vi "Size.vi"(7 "VI":refnum<vi>, 8 "Error":errorcluster, 9 "WkSpace":T1, 11 "(FPSZ)":refnum<class "FPSZ.lvclass">) -> (0 "Error Out":errorcluster, 3 "(FPSZ) Out":refnum<class "FPSZ.lvclass">, 5 "VI Out":refnum<vi>)   [LabVIEW 2020, in "FPSZ.lvclass"]
uses:
  FPSZ.lvclass
  <vilib>/Utility/miscctls.llb/LVRectTypeDef.ctl
  FPSZ.lvclass/FPSZ.ctl
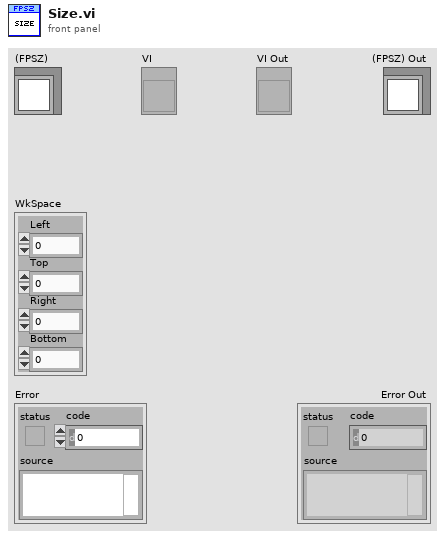
[diagram p1: front panel]
types:
  T1 = typedef "LVRectTypeDef.ctl" = cluster{"Left":i16, "Top":i16, "Right":i16, "Bottom":i16}
  T2 = typedef "LVPositionTypeDef.ctl" = cluster{"Left":i32, "Top":i32}
  T3 = typedef "LVBoundsTypeDef.ctl" = cluster{"Width":u32, "Height":u32}
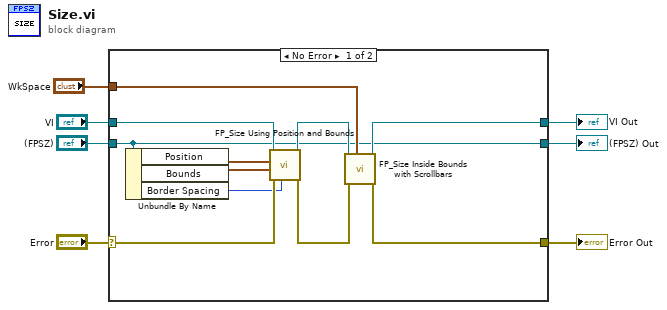
[diagram p0: block diagram]
diagram:
  n1 = case shown="No Error" "Error" {
    selector: "Error" -> [w18 w21]
    tunnel: [w12 w21] -> w6
    tunnel: [w8 w20] -> w4
    tunnel: "(FPSZ)" -> [w8 w20]
    tunnel: "VI" -> [w17 w19]
    tunnel: [w13 w19] -> w2
    tunnel: "WkSpace" -> [w14 _]
    frame No Error {
      n2 = Unbundle By Name(w8) -> ("Position"=w10:T2, "Bounds"=w9:T3, "Border Spacing"=w11:i16)
      n3 = call "FP_Size Using Position and Bounds.vi"("Border Spacing"=w11, "Error"=w18, "Bounds"=w9, "Position"=w10, "VI"=w17) -> ("Error Out"=w15:errorcluster, "VI Out"=w16:refnum<vi>)  [unwired: 4 in, 1 out]
      n4 = call "FP_Size Inside Bounds with Scrollbars.vi"("WkSpace"=w14, "Error"=w15, "VI"=w16) -> ("Error Out"=w12:errorcluster, "VI Out"=w13:refnum<vi>)  [unwired: 6 in, 1 out]
    }
    frame Error {
    }
  }
  "Error Out" <- w6
  "(FPSZ) Out" <- w4
  "VI Out" <- w2
